vi "VI Server.vi"() -> ()   [LabVIEW 2009]
doc: "This example shows how to use Command Line Arguments property node to launch a LabVIEW VI and pass user-defined arguments.\n\nUse the following syntax in the Command Line to launch this VI:\n\n\"<full path to LabVIEW directory>\\labview.exe\" \"<full path to LabVIEW directory>\\examples\\viserver\\cmdline.llb\\CommandLine.vi\"\n\nThis will launch CommandLine.vi\n\nThis VI is set to run when opened.\n\nAfter the VI name, enter two hyphens (--) surrounded by spaces before the user-defined arguments. \n\nThe arguments will be displayed in the front panel indicators.\n\nThe correct syntax for arguments that can be passed is\n/number:\n/boolean:\n/string:\nAfter (:) enter the appropriate value; a number, 0 or 1 boolean, a string.\n\nIf you enter more than one argument, they need to be separated with a space."
uses:
  <vilib>/Utility/miscctls.llb/LVRectTypeDef.ctl
panel:
  out "Version Number":u32
  out "Command Line Arguments":string[](array[string])
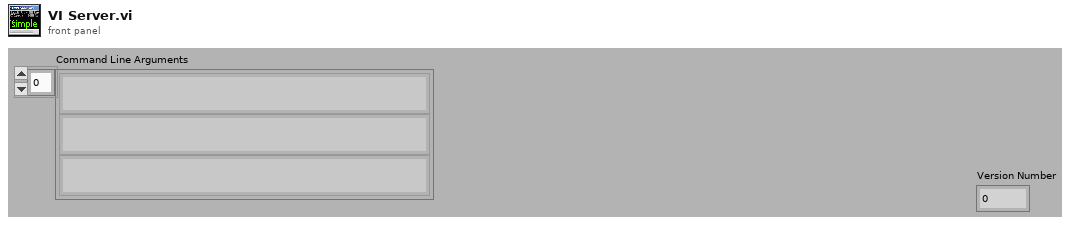
[diagram p1: front panel]
types:
  T1 = typedef "LVRectTypeDef.ctl" = cluster{"Left":i16, "Top":i16, "Right":i16, "Bottom":i16}
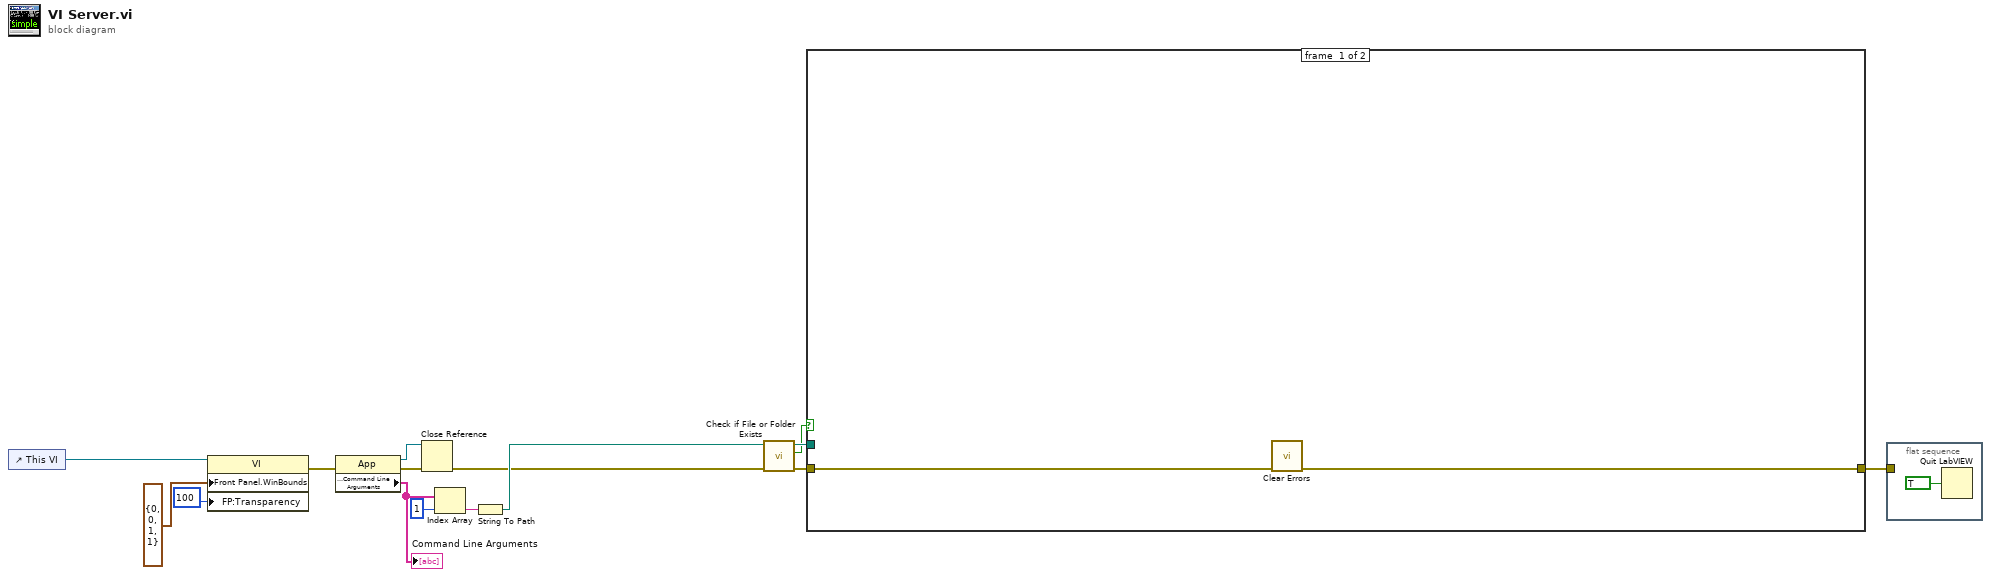
[diagram p0: block diagram]
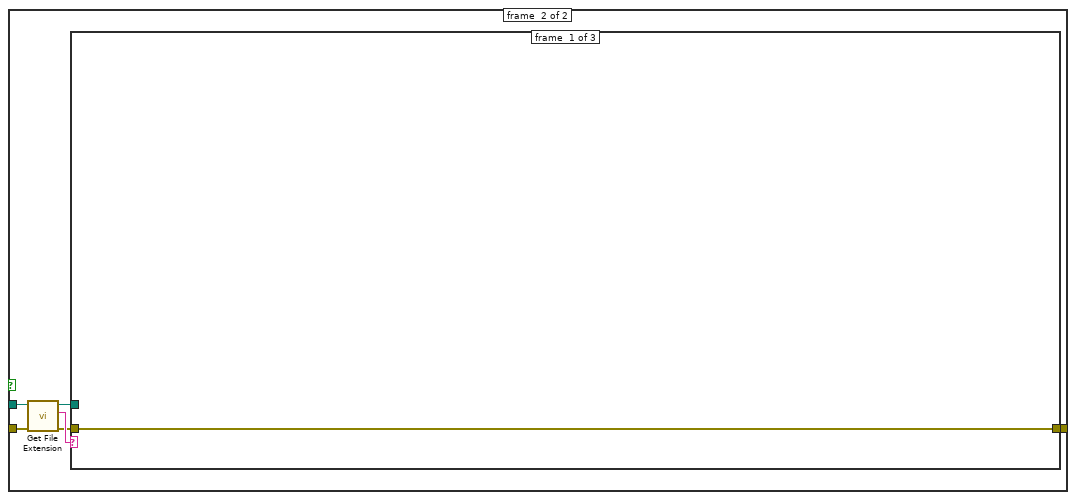
[diagram p2: hidden frame]
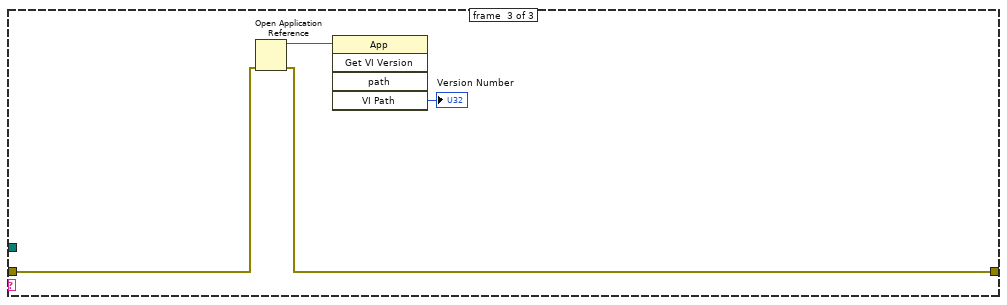
[diagram p4: hidden frame]
diagram:
  n1 = control-ref of="This VI"() -> (w10:refnum<vi>)
  n2 = property class="VI"(reference=w10, "Front Panel.WinBounds"=T1 {"Left"=0, "Top"=0, "Right"=1, "Bottom"=1} ("Front Panel Window:Window Bounds"), "FP:Transparency"=u8 100 ("Front Panel Window:Transparency")) -> (error out=w9:errorcluster)  [unwired: 1 in, 1 out]
  n3 = property class="App"(error in=w9) -> (reference out=w6:refnum<vi>, error out=w7:errorcluster, "Application:Command Line Arguments"=w5:string[])  [unwired: 1 in]
  "Command Line Arguments" <- w5
  n4 = Close Reference(reference=w6, error in (no error)=w7) -> (error out=w12:errorcluster)
  n5 = Index Array(array=w5, index=1) -> (element=w3:string)
  n6 = String To Path(string=w3) -> (path=w15:path)
  n7 = call <vilib>:"Check if File or Folder Exists.vi"("error in (no error)"=w12, "path"=w15) -> ("error out"=w11:errorcluster, "file or folder exists?"=w13:bool, "dup path"=w14:path)  [unwired: 7 in]
  n8 = case shown="True" w13 {
    tunnel: w14 -> [_ w21]
    tunnel: w11 -> [w17 w20]
    tunnel: [w16 w18] -> w8
    frame #0 {
      n9 = call <vilib>:"Clear Errors.vi"("error in (no error)"=w17) -> ("error out"=w16:errorcluster)  [unwired: 6 in]
    }
    frame #1 {
      n10 = call <vilib>:"Get File Extension.vi"("error in (no error)"=w20, "file"=w21) -> ("error out"=w19:errorcluster, "lowercase file extension"=w23:string, "dup file"=w22:path)  [unwired: 6 in, 1 out]
      n11 = case shown="\"vi\"" w23 {
        tunnel: w22 -> [_ _ _]
        tunnel: w19 -> [w24 w25 w27]
        tunnel: [w24 w25 w26] -> w18
        frame #0 {
        }
        frame #1 {
        }
        frame #2 {
          n12 = Open Application Reference(8:w27) -> (0:w26:errorcluster, 3:w29:refnum<vi>)  [unwired: 3 in]
          n13 = invoke class="App" method="Get VI Version"(reference=w29) -> ("VI Path"=→"Version Number":u32)  [unwired: 4 in, 4 out]
        }
      }
    }
  }
  n14 = flat-sequence {
    tunnel: w8 -> [_]
    frame #0 {
      n15 = Quit LabVIEW(quit? (T)=TRUE) -> ()
    }
  }
